vi "AnalogConfigWrite.vi"(8 "error in (no error)":errorcluster, 11 "AnalogConfig":T1) -> (0 "error out":errorcluster)   [LabVIEW 2020, in "Settings.lvlib"]
uses:
  Settings.lvlib
  Acquisition/AnalogConfig--cluster.ctl
  <vilib>/drjdpowell/SQLite Library/SQL Connection/Open (path).vi
  <vilib>/drjdpowell/SQLite Library/SQL Connection/Open (string).vi
  <vilib>/AdvancedString/Path To Command Line String.vi
  <vilib>/drjdpowell/SQLite Library/SQL Connection/Execute SQL (No results).vi
  <vilib>/drjdpowell/SQLite Library/SQL Connection/Connection.lvclass
  <vilib>/drjdpowell/SQLite Library/SQLite.lvlib
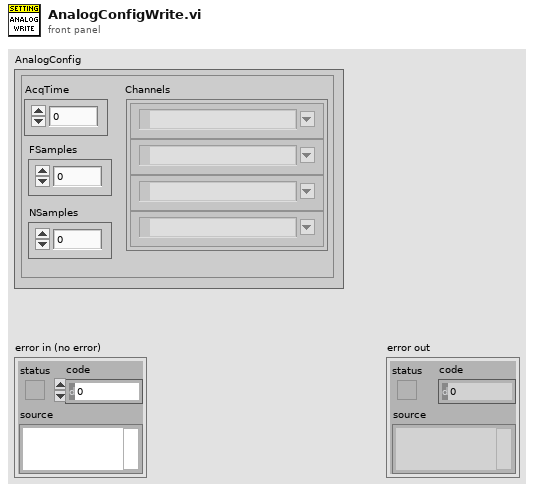
[diagram p1: front panel]
types:
  T1 = typedef "AnalogConfig--cluster.ctl" = cluster{"AcqTime":dbl, "FSamples":dbl, "NSamples":dbl, "Channels":tag[]}
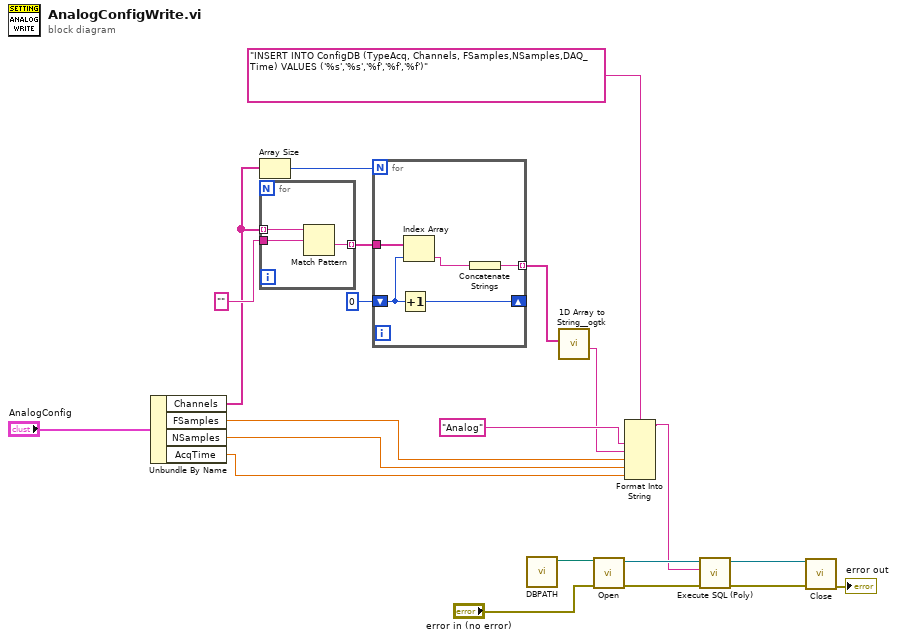
[diagram p0: block diagram]
diagram:
  n1 = Unbundle By Name("AnalogConfig") -> ("Channels"=w7:tag[], "FSamples"=w6:dbl, "NSamples"=w5:dbl, "AcqTime"=w4:dbl)
  n2 = Array Size(array=w7) -> (size(s)=w11:i32)
  n3 = for {
    tunnel: w7 -> [w24] mode=indexing
    tunnel: [w23] -> w10 mode=indexing
    tunnel: "" ("regular expression") -> [w22]
    n4 = Match Pattern(string=w24, regular expression=w22) -> (after substring=w23:string)  [unwired: 1 in, 3 out]
  }
  n5 = for {
    N: w11 -> [_]
    shift-right: [w27] -> _
    shift-left: 0 -> [w28]
    tunnel: w10 -> [w29]
    tunnel: [w25] -> w12 mode=indexing
    n6 = Increment(x=w28) -> (x+1=w27:i32)
    n7 = Index Array(array=w29, index=w28) -> (element=w26:string)
    n8 = Concatenate Strings(w26) -> (w25:string)
  }
  n9 = call "DBPATH.vi"() -> ("appended path"=w17:path)  [unwired: 11 in]
  n10 = call <userlib>:"1D Array to String__ogtk.vi"("Array of Strings"=w12) -> ("delimited string"=w2:string)  [unwired: 10 in]
  n11 = call-poly <vilib>:"Open.vi"("error in (no error)"="error in (no error)", "db file"=w17) -> ("error out"=w21:errorcluster, "SQLite Connection"=w19:refnum<class "Connection.lvclass">)  [unwired: 8 in]
  n12 = Format Into String(format string="INSERT INTO ConfigDB (TypeAcq, Channels, FSamples,NSamples,DAQ_Time) VALUES ('%s','%s','%f','%f','%f')", "Analog" ("input 1"), w2, w6, w5, w4) -> (resulting string=w14:string)  [unwired: 2 in, 1 out]
  n13 = call-poly <vilib>:"Execute SQL (Poly).vi"("error in (no error)"=w21, "SQL"=w14, "SQLite Connection in"=w19) -> ("error out"=w20:errorcluster, "SQLite Connection"=w18:refnum<class "Connection.lvclass">)  [unwired: 7 in]
  n14 = call-dynamic "Close.vi"("error in (no error)"=w20, "SQLite Connection in"=w18) -> ("error out"=→"error out":errorcluster)  [unwired: 9 in]
